vi "Set initial time.vi"(7 "DAQ":T1 {"Config"."Input Config" items=["default"=-1, "RSE"=10083, "NRSE"=10078, "Differential"=10106, "Pseudodifferential"=12529]}, 8 "error in":errorcluster) -> (0 "error out":errorcluster, 5 "DAQ out":T1 {"Config"."Input Config" items=["default"=-1, "RSE"=10083, "NRSE"=10078, "Differential"=10106, "Pseudodifferential"=12529]})   [LabVIEW 2017, in "DAQ.lvlib"]
uses:
  DAQ.lvlib
  Controls/Params.ctl
panel:
  out "time stamp":timestamp format="%<%I:%M %p\n%d/%m/%y>T"
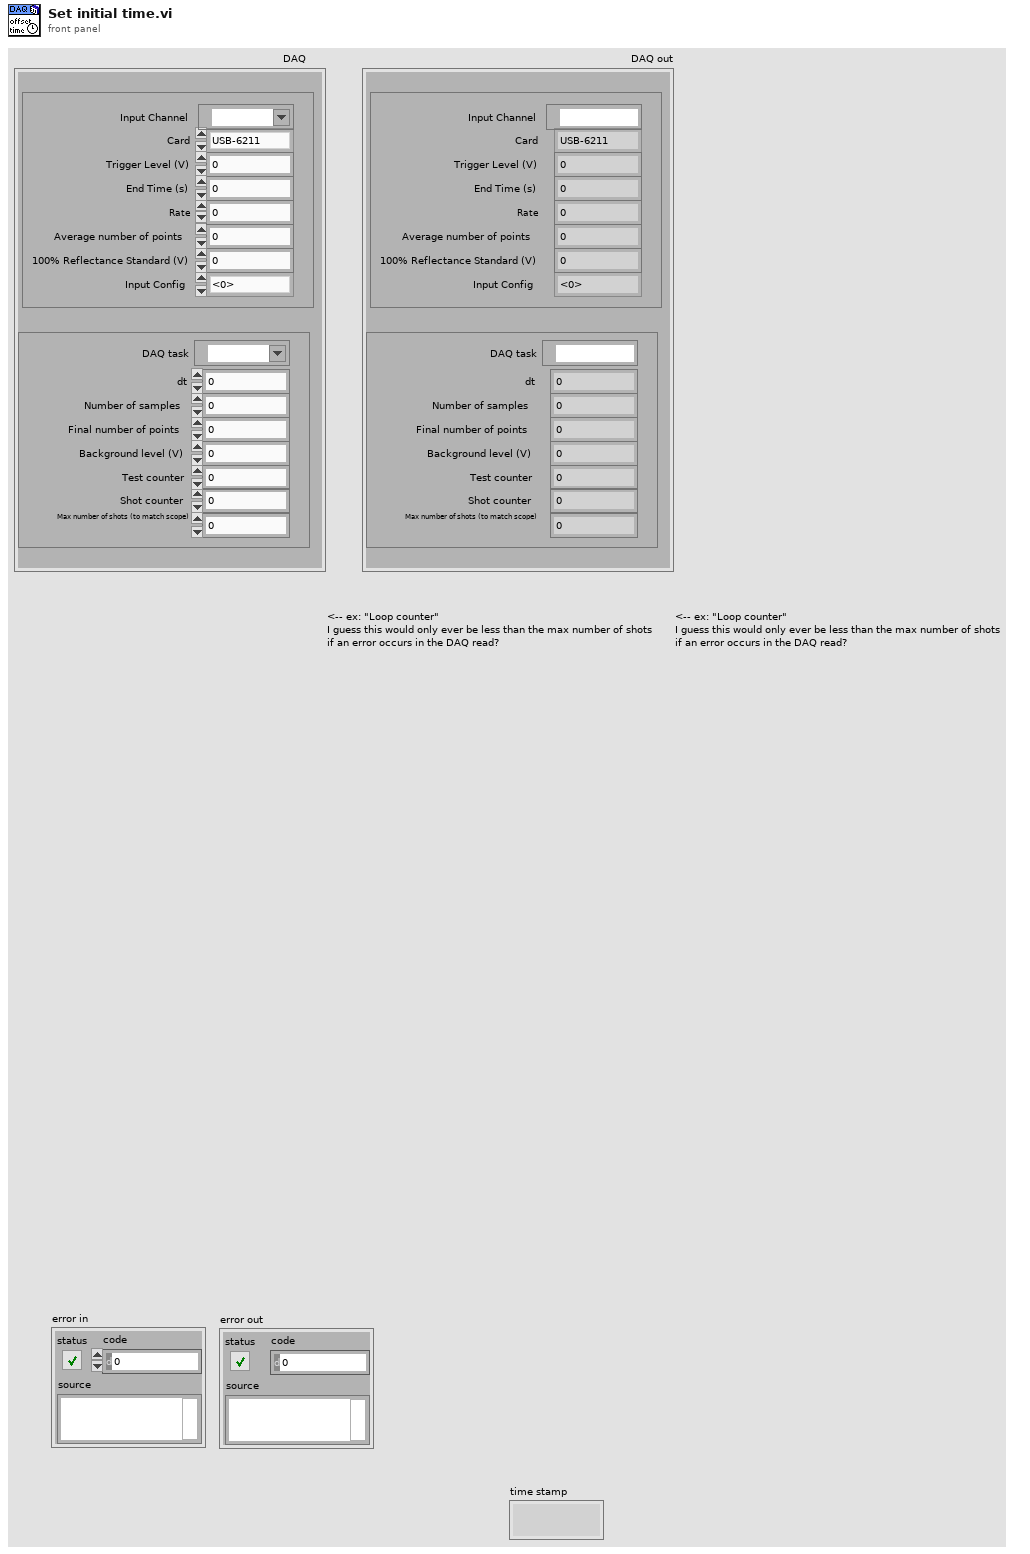
[diagram p1: front panel]
types:
  T1 = typedef "DAQ.lvlib/Params.ctl" = cluster{"Data":cluster{"Live":waveform(dbl), "Accumulated":waveform(dbl), "Averaged":waveform(dbl), "Final":waveform(dbl), "data array":dbl[], "live time array":dbl[], "DOD (final)":dbl[], "Live (decimated)":waveform(dbl)}, "Config":cluster{"Input Config":i32, "Card":enum16{"USB-6211", "USB-6251"}, "100% Reflectance Standard (V)":dbl, "Input Channel":tag, "Average number of points":dbl, "Trigger Level (V)":dbl, "Rate":i32, "End Time (s)":dbl}, "Indicators":cluster{"Final number of points":dbl, "Number of samples":dbl, "dt":dbl, "Max number of shots (to match scope)":i32, "Shot counter":i32, "Test counter":i32, "Background level (V)":dbl, "DAQ task":refnum<k21>}}
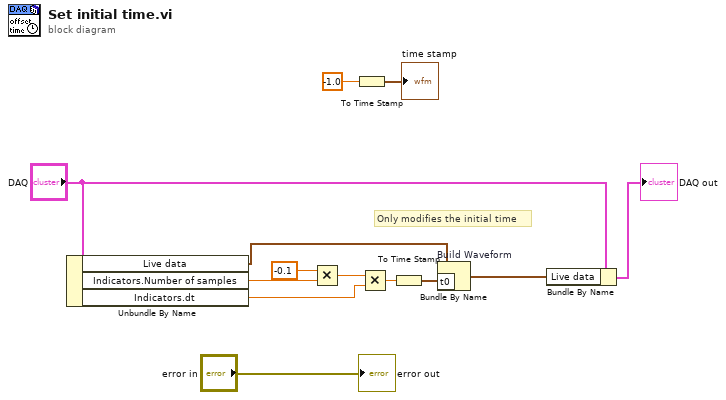
[diagram p0: block diagram]
diagram:
  # "Only modifies the initial time"
  n1 = Unbundle By Name("DAQ") -> ("Live data"=w3:waveform(dbl), "Indicators.Number of samples"=w12:dbl, "Indicators.dt"=w13:dbl)
  n2 = Multiply(x=-0.1 ("y"), y=w12) -> (x*y=w10:dbl)
  n3 = To Time Stamp(1:-1.0 ("number")) -> (0:→"time stamp":timestamp)
  n4 = Multiply(x=w10, y=w13) -> (x*y=w9:dbl)
  n5 = To Time Stamp(1:w9) -> (0:w8:timestamp)
  n6 = Bundle By Name "Build Waveform"(cluster=w3, "t0"=w8) -> (w5:waveform(dbl))
  n7 = Bundle By Name(cluster="DAQ", "Live data"=w5) -> (→"DAQ out":T1)
  "error out" <- "error in"
